vi "LinearSystemLoop_DCMotor_Pack_Ctrl.vi"(4 "Max Ctrl Out V":dbl=12.0, 6 "Pos Ctrl Tol Rad":dbl=90000000000.0, 7 "Vel Model Std Dev Rad/Sec":dbl=0.1, 8 "Vel Ctrl Tol Rad/Sec":dbl=0.04, 9 "Pos Meas Std Dev Rad":dbl=9000.0, 10 "Vel Meas Std Dev Rad/Sec":dbl=0.02, 11 "Pos Model Std Dev Rad":dbl=0.8) -> (3 "LinearSystemLoop_DCMotor_Ctrl_Params":T1={"Vel Model Std Dev Rad/Sec"=0.0, "Vel Meas Std Dev Rad/Sec"=0.0, "Vel Ctrl Tol Rad/Sec"=0.0, "Max Ctrl Out V"=0.0, "Pos Model Std Dev Rad"=0.8, "Pos Meas Std Dev Rad"=0.02, "Pos Ctrl Tol Rad"=0.8})   [LabVIEW 2019, in "Trajectory_Library.lvlib"]
uses:
  TypeDef/LINEAR_SYSTEM_LOOP_DCMOTOR_CTRL_PARAMS.ctl
  Trajectory_Library.lvlib
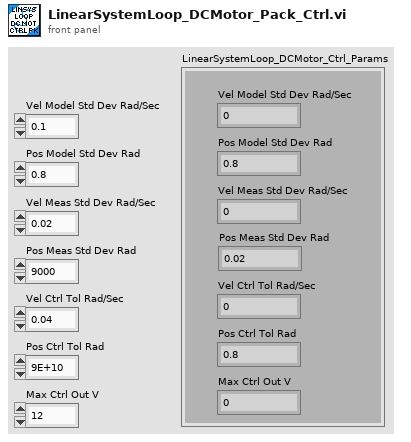
[diagram p1: front panel]
types:
  T1 = typedef "Trajectory_Library.lvlib/LINEAR_SYSTEM_LOOP_DCMOTOR_CTRL_PARAMS.ctl" = cluster{"Vel Model Std Dev Rad/Sec":dbl, "Vel Meas Std Dev Rad/Sec":dbl, "Vel Ctrl Tol Rad/Sec":dbl, "Max Ctrl Out V":dbl, "Pos Model Std Dev Rad":dbl, "Pos Meas Std Dev Rad":dbl, "Pos Ctrl Tol Rad":dbl}
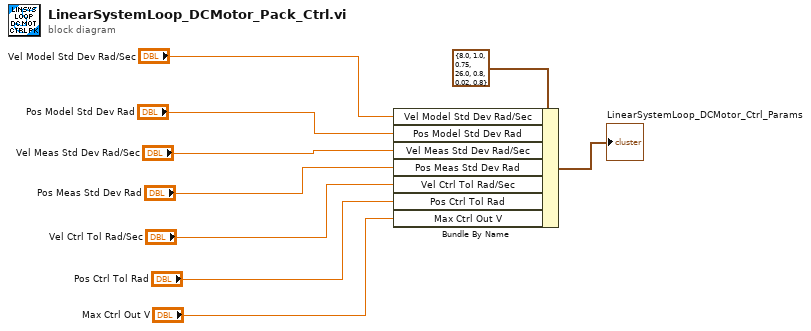
[diagram p0: block diagram]
diagram:
  n1 = Bundle By Name(cluster=T1 {"Vel Model Std Dev Rad/Sec"=8.0, "Vel Meas Std Dev Rad/Sec"=1.0, "Vel Ctrl Tol Rad/Sec"=0.75, "Max Ctrl Out V"=26.0, "Pos Model Std Dev Rad"=0.8, "Pos Meas Std Dev Rad"=0.02, "Pos Ctrl Tol Rad"=0.8} ("DCMotorSim_Model _Params"), "Vel Model Std Dev Rad/Sec"="Vel Model Std Dev Rad/Sec", "Pos Model Std Dev Rad"="Pos Model Std Dev Rad", "Vel Meas Std Dev Rad/Sec"="Vel Meas Std Dev Rad/Sec", "Pos Meas Std Dev Rad"="Pos Meas Std Dev Rad", "Vel Ctrl Tol Rad/Sec"="Vel Ctrl Tol Rad/Sec", "Pos Ctrl Tol Rad"="Pos Ctrl Tol Rad", "Max Ctrl Out V"="Max Ctrl Out V") -> (→"LinearSystemLoop_DCMotor_Ctrl_Params":T1)
